vi "niScope Configure Vertical.vi"(0 "instrument handle":refnum<k15>, 1 "probe attenuation":dbl=1.0 format="%.1f", 2 "vertical coupling":T1=1 items=["AC", "DC", "Ground"], 5 "channels":string="0", 7 "vertical range":dbl=10.0 format="%.2f", 9 "vertical offset":dbl format="%.4f", 11 "error in":errorcluster, 12 "channel enabled":bool=TRUE) -> (4 "instrument handle out":refnum<k15>, 15 "error out":errorcluster)   [LabVIEW 2020]
doc: "Configures the most commonly configured properties of the digitizer vertical subsystem, such as the range, offset, coupling, probe attenuation, and the channel name."
uses:
  niScope vertical coupling.ctl
  niScope_32.dll
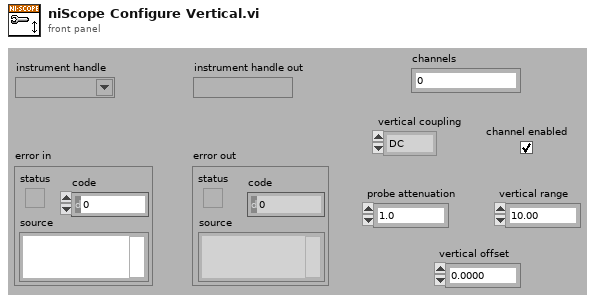
[diagram p1: front panel]
types:
  T1 = typedef "niScope vertical coupling.ctl" = i32
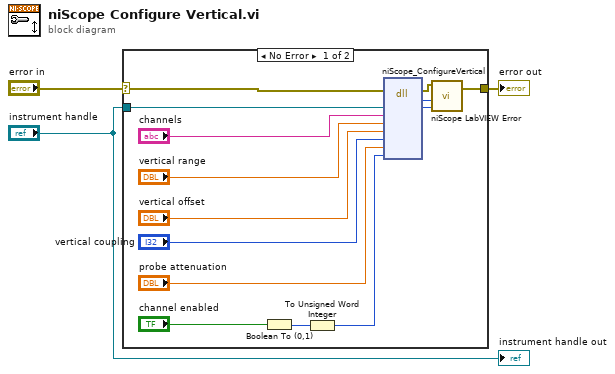
[diagram p0: block diagram]
diagram:
  n1 = case shown="No Error" "error in" {
    selector: "error in" -> [w5 w18]
    tunnel: [w7 w18] -> w2
    tunnel: "instrument handle" -> [w17 _]
    frame No Error {
      n2 = Boolean To (0,1)(Boolean="channel enabled") -> (0, 1=w11:i16)
      n3 = To Unsigned Word Integer(number=w11) -> (unsigned 16bit integer=w10:u16)
      n4 = dll-call lib="niScope_*.*" fn="niScope_ConfigureVertical"(error in=w5, "instrument handle"=w17, "channel"="channels", "range"="vertical range", "offset"="vertical offset", "coupling"="vertical coupling", "probeAttenuation"="probe attenuation", "enabled"=w10) -> (error out=w4:errorcluster, "status"=w9:i32, "instrument handle"=w8:u32)  [unwired: 8 in, 1 out]
      n5 = call "niScope LabVIEW Error.vi"("instrument handle"=w8, "niScope error code (0)"=w9, "error in (no error)"=w4) -> ("error out"=w7:errorcluster)  [unwired: 2 in]
    }
    frame Error {
    }
  }
  "error out" <- w2
  "instrument handle out" <- "instrument handle"
